vi "Initial_Binarization_Settings-2.vi"() -> (0 "Binarization Settings":cluster{"MinBin2":sgl, "MaxBin2":sgl}[](array[cluster]))   [LabVIEW 2013]
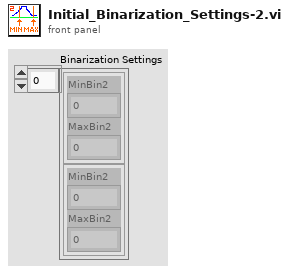
[diagram p1: front panel]
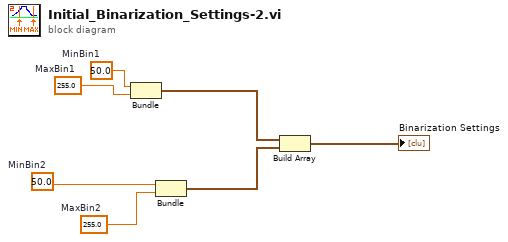
[diagram p0: block diagram]
diagram:
  w4 = sgl 255.0  # MaxBin2
  w5 = sgl 50.0  # MinBin2
  w6 = sgl 255.0  # MaxBin1
  w7 = sgl 50.0  # MinBin1
  n1 = Bundle("MinBin1"=w7, "MaxBin1"=w6) -> (w3:cluster{"MinBin1":sgl, "MaxBin1":sgl})  [unwired: 1 in]
  n2 = Bundle("MinBin2"=w5, "MaxBin2"=w4) -> (w2:cluster{"MinBin2":sgl, "MaxBin2":sgl})  [unwired: 1 in]
  n3 = Build Array(w3, w2) -> (→"Binarization Settings":cluster{"MinBin2":sgl, "MaxBin2":sgl}[])
